vi "subVIcreateChannel.vi"(0 "maximum value":dbl=5.0 format="%0.2f", 1 "name to assign":string, 2 "minimum value":dbl=-5.0 format="%0.2f", 3 "input terminal configuration":i32(ring)=-1 items=["Default"=-1, "RSE"=10083, "NRSE"=10078, "Differential"=10106, "Pseudodifferential"=12529], 4 "physical channels":tag, 5 "units":i32(ring)=10348 items=["Volts"=10348, "From Custom Scale"=10065], 6 "error in":errorcluster) -> (7 "data":dbl format="%0.2f", 8 "error out":errorcluster)   [LabVIEW 2015]
doc: "Create a channel for DAQ and read data from the channel.\n\nInputs:\n======\nmaximum value,\nmanimum value,\nunits,\nInput terminal configuration,\nname to assign,\nphysical channels,\nerror in.\n\noutputs:\n=======\ndata,\nerror out."
uses:
  <vilib>/DAQmx/read.llb/DAQmx Read (Analog DBL 1Chan 1Samp).vi
  <vilib>/DAQmx/create/channels.llb/DAQmx Create Channel (AI-Voltage-Basic).vi
  <vilib>/DAQmx/miscellaneous.llb/DAQmx Fill In Error Info.vi
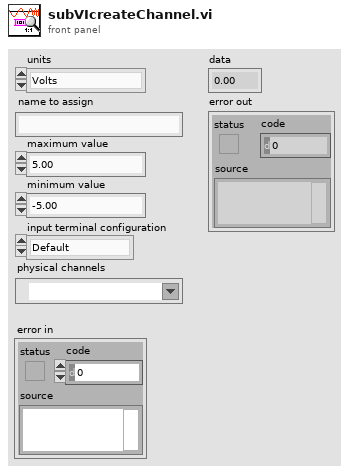
[diagram p1: front panel]
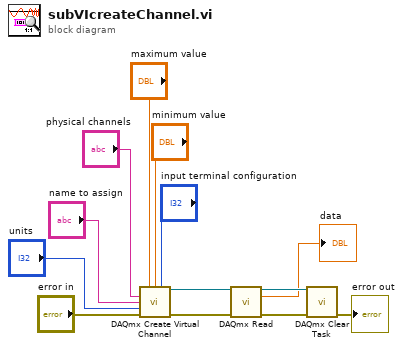
[diagram p0: block diagram]
diagram:
  n1 = call-poly <vilib>:"DAQmx Create Virtual Channel.vi"("maximum value"="maximum value", "minimum value"="minimum value", "input terminal configuration"="input terminal configuration", "physical channels"="physical channels", "name to assign"="name to assign", "units"="units", "error in"="error in") -> ("task out"=w13:refnum<k21>, "error out"=w11:errorcluster)  [unwired: 7 in]
  n2 = call-poly <vilib>:"DAQmx Read.vi"("task/channels in"=w13, "error in"=w11) -> ("task out"=w12:refnum<k21>, "data"=→"data":dbl, "error out"=w10:errorcluster)  [unwired: 11 in]
  n3 = call <vilib>:"DAQmx Clear Task.vi"("task in"=w12, "error in"=w10) -> ("error out"=→"error out":errorcluster)  [unwired: 13 in]
